vi "_clear_header_maps.vi"(11 "httpHeaders in":refnum<class "httpHeaders.lvclass">) -> (3 "httpHeaders out":refnum<class "httpHeaders.lvclass">)   [LabVIEW 2020, in "httpClient.lvlib" / "httpHeaders.lvclass"]
uses:
  httpHeaders.lvclass
  httpHeaders.lvclass/httpHeaders.ctl
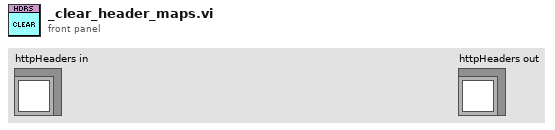
[diagram p1: front panel]
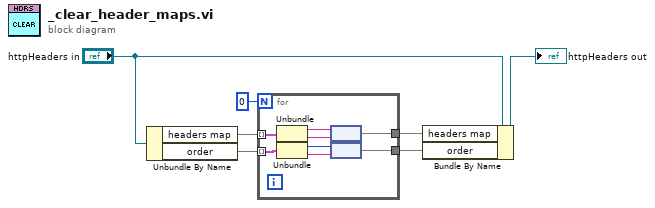
[diagram p0: block diagram]
diagram:
  n1 = Unbundle By Name("httpHeaders in") -> ("headers map"=w4:map{string, string}, "order"=w3:map{i32, string})
  n2 = for {
    N: 0 -> [_]
    tunnel: w4 -> [w11] mode=indexing
    tunnel: w3 -> [w10] mode=indexing
    tunnel: [w9] -> w2
    tunnel: [w8] -> w1
    n3 = Unbundle(w11) -> ("key"=w15:string, "value"=w14:string)
    n4 = Unbundle(w10) -> ("index"=w12:i32, "key"=w13:string)
    n5 = node(w15, w14) -> (w9:map{string, string})
    n6 = node(w12, w13) -> (w8:map{i32, string})
  }
  n7 = Bundle By Name(cluster="httpHeaders in", "headers map"=w2, "order"=w1) -> (→"httpHeaders out":refnum<class "httpHeaders.lvclass">)
